vi "test Export SLSC-12252.vi"(8 "error in (no error)":errorcluster, 11 "TestCase in":refnum<class "SLSC Switch Export Unit Tests.lvclass">) -> (0 "error out":errorcluster, 3 "TestCase out":refnum<class "SLSC Switch Export Unit Tests.lvclass">)   [LabVIEW 2017, in "SLSC Switch Export Unit Tests.lvclass"]
uses:
  SLSC Switch Export Unit Tests.lvclass
  <vilib>/NI/NI VeriStand Advanced SysDef API/_Types/SysDef.Export.ctl
  <vilib>/NI/NI VeriStand Advanced SysDef API/_Types/TreeItem.ctl
  <vilib>/NI/NI VeriStand Advanced SysDef API/_Types/TreeItem.Info.ctl
  <vilib>/NI Veristand/Custom Device API/Custom Device Channel.ctl
  <vilib>/NI Veristand/Custom Device API/Custom Device Channel Type.ctl
  <vilib>/NI Veristand/Custom Device API/Custom Device Waveform.ctl
  <vilib>/NI Veristand/Custom Device API/Custom Device Waveform DataType.ctl
  <vilib>/NI/NI VeriStand Advanced SysDef API/_Types/TreeItem.Property.ctl
  SLSC Switch Export Unit Tests.lvclass/SLSC Switch Export Unit Tests.ctl
  <vilib>/addons/_JKI Toolkits/VI Tester/TestCase.llb/TestCase.lvclass
  Scripting/SLSC Switch Scripting.lvlib
  <vilib>/NI/NI VeriStand Custom Device Import and Export Tool/ImportExport.lvlib
  <vilib>/NI/NI VeriStand Advanced SysDef API/SysDef API/Advanced System Definition.lvlib
  <vilib>/NI Veristand/Custom Device API/Custom Device API.lvlib
  C:/Program Files (x86)/National Instruments/LabVIEW 2017/vi.lib/addons/_JKI Toolkits/VI Tester/TestCase.llb/TestCase.lvclass
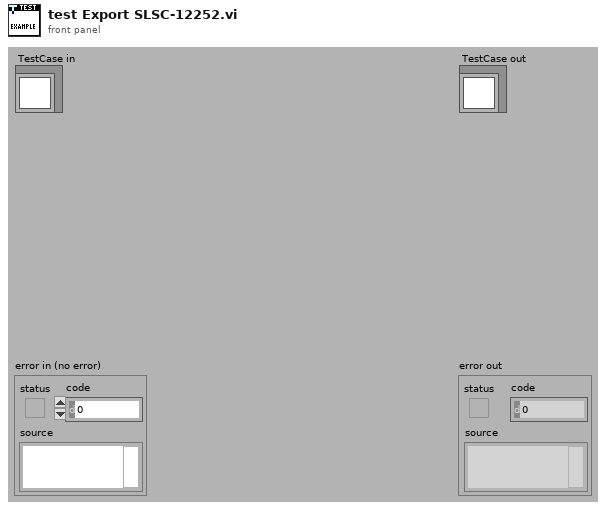
[diagram p1: front panel]
types:
  T1 = typedef "Advanced System Definition.lvlib/SysDef.Export.ctl" = cluster{"Version":string, "Tree":T2[]}
  T2 = typedef "Advanced System Definition.lvlib/TreeItem.ctl" = cluster{"Item Info":T3, "Parent Path":string[], "Properties":T8[]}
  T3 = typedef "Advanced System Definition.lvlib/TreeItem.Info.ctl" = cluster{"Name":string, "Description":string, "GUID":string, "Is Channel":bool, "Channel":T4, "Is Waveform":bool, "Waveform":T6}
  T4 = typedef "Custom Device API.lvlib/Custom Device Channel.ctl" = cluster{"Type":T5, "Units":string, "Default Value":dbl, "Faultable":bool, "Scalable":bool}
  T5 = typedef "Custom Device API.lvlib/Custom Device Channel Type.ctl" = enum16{"Input", "Output"}
  T6 = typedef "Custom Device API.lvlib/Custom Device Waveform.ctl" = cluster{"Data Type":T7, "Units":string}
  T7 = typedef "Custom Device API.lvlib/Custom Device Waveform DataType.ctl" = enum16{"Double", "Complex Double"}
  T8 = typedef "Advanced System Definition.lvlib/TreeItem.Property.ctl" = cluster{"Name":string, "Type":i32, "Value":variant}
  T9 = typedef "Custom Device API.lvlib/Custom Device Item Ref.ctl" = u64
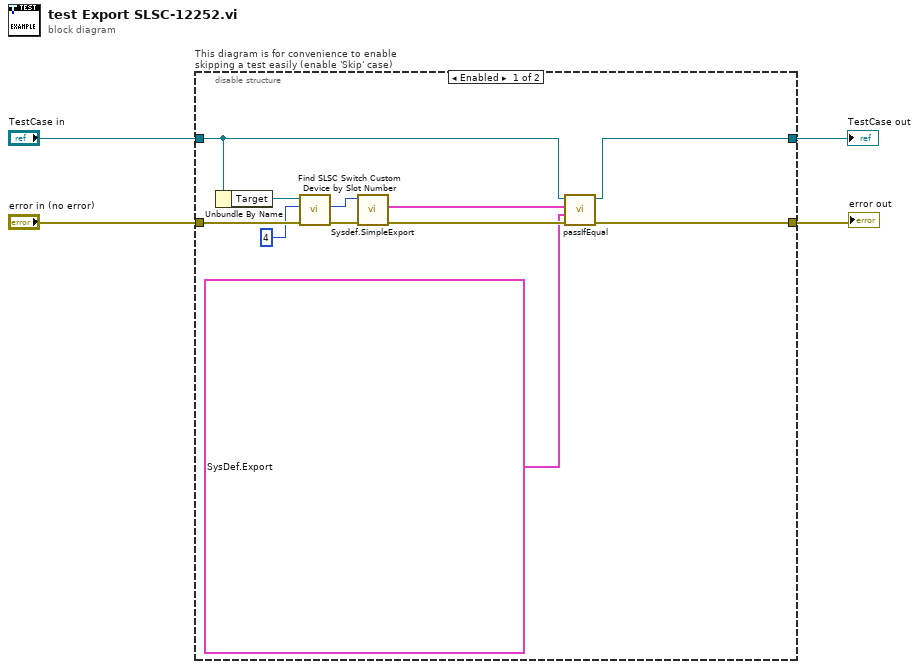
[diagram p0: block diagram]
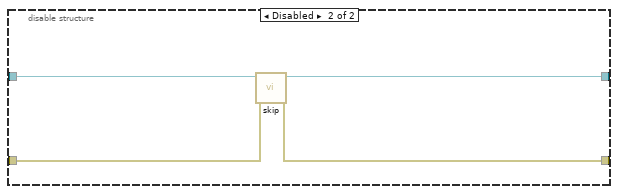
[diagram p2: hidden frame]
diagram:
  n1 = disable-structure "This diagram is for convenience to enable skipping a test easily (enable 'Skip' case)" shown="Enabled" {
    disable-tunnel: "TestCase in" -> [w7 w19]
    disable-tunnel: [w6 w17] -> w1
    disable-tunnel: [w9 w18] -> w3
    disable-tunnel: "error in (no error)" -> [w15 w16]
    frame Enabled {
      n2 = Unbundle By Name(w7) -> ("Target"=w14:refnum<k24>)
      n3 = call "Find SLSC Switch Custom Device by Slot Number.vi"("error in (no error)"=w15, "slot number"=u32 4, "Target in"=w14) -> ("error out"=w12:errorcluster, "SLSC Switch Custom Device Ref"=w11:T9)  [unwired: 6 in, 1 out]
      n4 = call <vilib>:"Sysdef.SimpleExport.vi"("error in (no error)"=w12, "ID"=w11) -> ("error out"=w10:errorcluster, "Export"=w8:T1)  [unwired: 7 in, 1 out]
      n5 = call-dynamic "passIfEqual.vi"("error in (no error)"=w10, "y"=T1 {"Version"="1.0.0", "Tree"=[{"Item Info"={"Name"="Slot 4 (SLSC Switch)", "Description"="", "GUID"="5e47c8de-3ec6-490b-8897-5526d4aea756", "Is Channel"=FALSE, "Channel"={"Type"=enum."Input", "Units"="", "Default Value"=0.0, "Faultable"=FALSE, "Scalable"=FALSE}, "Is Waveform"=FALSE, "Waveform"={"Data Type"=enum."Double", "Units"=""}}, "Parent Path"=["Targets", "Controller", "Hardware", "SLSC", "SLSC Chassis", "Modules"], "Properties"=[{"Name"="user.CD.Routing and Faulting.API Version", "Type"=3, "Value"=variant(u32 1)}, {"Name"="user.CD.Model", "Type"=0, "Value"=variant(string "SLSC-12252", "IsBinary"=variant(bool FALSE))}, {"Name"="user.CD.Routing and Faulting.Resource", "Type"=0, "Value"=variant(string "slsc-12001-0314b282-Mod4", "IsBinary"=variant(bool FALSE))}, {"Name"="user.CD.Topology", "Type"=0, "Value"=variant(string "NI12252_topology", "IsBinary"=variant(bool FALSE))}, {"Name"="user.CD.Capabilities", "Type"=0, "Value"=variant(string "{\"switchesSpecVersion\":1,\"switchesSpecOldestCompatibleVersion\":1,\"relays\":[{\"name\":\"Ch0\",\"actions\":[{\"type\":\"property\",\"resource\":\"Channel_0\",\"value\":\"NI.FIU.Preset.Load\"},{\"type\":\"command\",\"resource\":\"\",\"value\":\"NI.FIU.Update\"}]},{\"name\":\"Ch1\",\"actions\":[{\"type\":\"property\",\"resource\":\"Channel_1\",\"value\":\"NI.FIU.Preset.Load\"},{\"type\":\"command\",\"resource\":\"\",\"value\":\"NI.FIU.Update\"}]},{\"name\":\"Ch2\",\"actions\":[{\"type\":\"property\",\"resource\":\"Channel_2\",\"value\":\"NI.FIU.Preset.Load\"},{\"type\":\"command\",\"resource\":\"\",\"value\":\"NI.FIU.Update\"}]},{\"name\":\"Ch3\",\"actions\":[{\"type\":\"property\",\"resource\":\"Channel_3\",\"value\":\"NI.FIU.Preset.Load\"},{\"type\":\"command\",\"resource\":\"\",\"value\":\"NI.FIU.Update\"}]},{\"name\":\"Ch4\",\"actions\":[{\"type\":\"property\",\"resource\":\"Channel_4\",\"value\":\"NI.FIU.Preset.Load\"},{\"type\":\"command\",\"resource\":\"\",\"value\":\"NI.FIU.Update\"}]},{\"name\":\"Ch5\",\"actions\":[{\"type\":\"property\",\"resource\":\"Channel_5\",\"value\":\"NI.FIU.Preset.Load\"},{\"type\":\"command\",\"resource\":\"\",\"value\":\"NI.FIU.Update\"}]},{\"name\":\"Ch6\",\"actions\":[{\"type\":\"property\",\"resource\":\"Channel_6\",\"value\":\"NI.FIU.Preset.Load\"},{\"type\":\"command\",\"resource\":\"\",\"value\":\"NI.FIU.Update\"}]},{\"name\":\"Ch7\",\"actions\":[{\"type\":\"property\",\"resource\":\"Channel_7\",\"value\":\"NI.FIU.Preset.Load\"},{\"type\":\"command\",\"resource\":\"\",\"value\":\"NI.FIU.Update\"}]},{\"name\":\"Ch0_Ch1\",\"actions\":[{\"type\":\"property\",\"resource\":\"ChannelPair_0\",\"value\":\"NI.FIU.Preset.InterChannel\"},{\"type\":\"command\",\"resource\":\"\",\"value\":\"NI.FIU.Update\"}]},{\"name\":\"Ch2_Ch3\",\"actions\":[{\"type\":\"property\",\"resource\":\"ChannelPair_1\",\"value\":\"NI.FIU.Preset.InterChannel\"},{\"type\":\"command\",\"resource\":\"\",\"value\":\"NI.FIU.Update\"}]},{\"name\":\"Ch4_Ch5\",\"actions\":[{\"type\":\"property\",\"resource\":\"ChannelPair_2\",\"value\":\"NI.FIU.Preset.InterChannel\"},{\"type\":\"command\",\"resource\":\"\",\"value\":\"NI.FIU.Update\"}]},{\"name\":\"Ch6_Ch7\",\"actions\":[{\"type\":\"property\",\"resource\":\"ChannelPair_3\",\"value\":\"NI.FIU.Preset.InterChannel\"},{\"type\":\"command\",\"resource\":\"\",\"value\":\"NI.FIU.Update\"}]}],\"multiStateRelays\":[{\"name\":\"Ch0_Bus\",\"relays\":[{\"name\":\"Ch0_BusA\",\"actions\":[{\"type\":\"property\",\"resource\":\"Channel_0\",\"value\":\"NI.FIU.Preset.BusSource\",\"close\":1},{\"type\":\"command\",\"resource\":\"\",\"value\":\"NI.FIU.Update\"}]},{\"name\":\"Ch0_BusB\",\"actions\":[{\"type\":\"property\",\"resource\":\"Channel_0\",\"value\":\"NI.FIU.Preset.BusSource\",\"close\":2},{\"type\":\"command\",\"resource\":\"\",\"value\":\"NI.FIU.Update\"}]}]},{\"name\":\"Ch1_Bus\",\"relays\":[{\"name\":\"Ch1_BusA\",\"actions\":[{\"type\":\"property\",\"resource\":\"Channel_1\",\"value\":\"NI.FIU.Preset.BusSource\",\"close\":1},{\"type\":\"command\",\"resource\":\"\",\"value\":\"NI.FIU.Update\"}]},{\"name\":\"Ch1_BusB\",\"actions\":[{\"type\":\"property\",\"resource\":\"Channel_1\",\"value\":\"NI.FIU.Preset.BusSource\",\"close\":2},{\"type\":\"command\",\"resource\":\"\",\"value\":\"NI.FIU.Update\"}]}]},{\"name\":\"Ch2_Bus\",\"relays\":[{\"name\":\"Ch2_BusA\",\"actions\":[{\"type\":\"property\",\"resource\":\"Channel_2\",\"value\":\"NI.FIU.Preset.BusSource\",\"close\":1},{\"type\":\"command\",\"resource\":\"\",\"value\":\"NI.FIU.Update\"}]},{\"name\":\"Ch2_BusB\",\"actions\":[{\"type\":\"property\",\"resource\":\"Channel_2\",\"value\":\"NI.FIU.Preset.BusSource\",\"close\":2},{\"type\":\"command\",\"resource\":\"\",\"value\":\"NI.FIU.Update\"}]}]},{\"name\":\"Ch3_Bus\",\"relays\":[{\"name\":\"Ch3_BusA\",\"actions\":[{\"type\":\"property\",\"resource\":\"Channel_3\",\"value\":\"NI.FIU.Preset.BusSource\",\"close\":1},{\"type\":\"command\",\"resource\":\"\",\"value\":\"NI.FIU.Update\"}]},{\"name\":\"Ch3_BusB\",\"actions\":[{\"type\":\"property\",\"resource\":\"Channel_3\",\"value\":\"NI.FIU.Preset.BusSource\",\"close\":2},{\"type\":\"command\",\"resource\":\"\",\"value\":\"NI.FIU.Update\"}]}]},{\"name\":\"Ch4_Bus\",\"relays\":[{\"name\":\"Ch4_BusA\",\"actions\":[{\"type\":\"property\",\"resource\":\"Channel_4\",\"value\":\"NI.FIU.Preset.BusSource\",\"close\":1},{\"type\":\"command\",\"resource\":\"\",\"value\":\"NI.FIU.Update\"}]},{\"name\":\"Ch4_BusB\",\"actions\":[{\"type\":\"property\",\"resource\":\"Channel_4\",\"value\":\"NI.FIU.Preset.BusSource\",\"close\":2},{\"type\":\"command\",\"resource\":\"\",\"value\":\"NI.FIU.Update\"}]}]},{\"name\":\"Ch5_Bus\",\"relays\":[{\"name\":\"Ch5_BusA\",\"actions\":[{\"type\":\"property\",\"resource\":\"Channel_5\",\"value\":\"NI.FIU.Preset.BusSource\",\"close\":1},{\"type\":\"command\",\"resource\":\"\",\"value\":\"NI.FIU.Update\"}]},{\"name\":\"Ch5_BusB\",\"actions\":[{\"type\":\"property\",\"resource\":\"Channel_5\",\"value\":\"NI.FIU.Preset.BusSource\",\"close\":2},{\"type\":\"command\",\"resource\":\"\",\"value\":\"NI.FIU.Update\"}]}]},{\"name\":\"Ch6_Bus\",\"relays\":[{\"name\":\"Ch6_BusA\",\"actions\":[{\"type\":\"property\",\"resource\":\"Channel_6\",\"value\":\"NI.FIU.Preset.BusSource\",\"close\":1},{\"type\":\"command\",\"resource\":\"\",\"value\":\"NI.FIU.Update\"}]},{\"name\":\"Ch6_BusB\",\"actions\":[{\"type\":\"property\",\"resource\":\"Channel_6\",\"value\":\"NI.FIU.Preset.BusSource\",\"close\":2},{\"type\":\"command\",\"resource\":\"\",\"value\":\"NI.FIU.Update\"}]}]},{\"name\":\"Ch7_Bus\",\"relays\":[{\"name\":\"Ch7_BusA\",\"actions\":[{\"type\":\"property\",\"resource\":\"Channel_7\",\"value\":\"NI.FIU.Preset.BusSource\",\"close\":1},{\"type\":\"command\",\"resource\":\"\",\"value\":\"NI.FIU.Update\"}]},{\"name\":\"Ch7_BusB\",\"actions\":[{\"type\":\"property\",\"resource\":\"Channel_7\",\"value\":\"NI.FIU.Preset.BusSource\",\"close\":2},{\"type\":\"command\",\"resource\":\"\",\"value\":\"NI.FIU.Update\"}]}]}],\"topologies\":[{\"name\":\"NI12252_topology\",\"initialState\":{\"open\":[\"Ch0\",\"Ch0_BusA\",\"Ch0_BusB\",\"Ch1\",\"Ch1_BusA\",\"Ch1_BusB\",\"Ch2\",\"Ch2_BusA\",\"Ch2_BusB\",\"Ch3\",\"Ch3_BusA\",\"Ch3_BusB\",\"Ch4\",\"Ch4_BusA\",\"Ch4_BusB\",\"Ch5\",\"Ch5_BusA\",\"Ch5_BusB\",\"Ch6\",\"Ch6_BusA\",\"Ch6_BusB\",\"Ch7\",\"Ch7_BusA\",\"Ch7_BusB\",\"Ch0_Ch1\",\"Ch2_Ch3\",\"Ch4_Ch5\",\"Ch6_Ch7\"],\"close\":[]},\"channelList\":{\"names\":[\"DUT_Ch0\",\"LOAD_Ch0\",\"DUT_Ch1\",\"LOAD_Ch1\",\"DUT_Ch2\",\"LOAD_Ch2\",\"DUT_Ch3\",\"LOAD_Ch3\",\"DUT_Ch4\",\"LOAD_Ch4\",\"DUT_Ch5\",\"LOAD_Ch5\",\"DUT_Ch6\",\"LOAD_Ch6\",\"DUT_Ch7\",\"LOAD_Ch7\",\"BusA\",\"BusB\"]},\"connectionList\":[{\"src\":\"DUT_Ch0\",\"dest\":\"LOAD_Ch0\",\"relays\":[\"Ch0\"]},{\"src\":\"DUT_Ch0\",\"dest\":\"BusA\",\"relays\":[\"Ch0_BusA\"]},{\"src\":\"DUT_Ch0\",\"dest\":\"BusB\",\"relays\":[\"Ch0_BusB\"]},{\"src\":\"DUT_Ch1\",\"dest\":\"LOAD_Ch1\",\"relays\":[\"Ch1\"]},{\"src\":\"DUT_Ch1\",\"dest\":\"BusA\",\"relays\":[\"Ch1_BusA\"]},{\"src\":\"DUT_Ch1\",\"dest\":\"BusB\",\"relays\":[\"Ch1_BusB\"]},{\"src\":\"DUT_Ch2\",\"dest\":\"LOAD_Ch2\",\"relays\":[\"Ch2\"]},{\"src\":\"DUT_Ch2\",\"dest\":\"BusA\",\"relays\":[\"Ch2_BusA\"]},{\"src\":\"DUT_Ch2\",\"dest\":\"BusB\",\"relays\":[\"Ch2_BusB\"]},{\"src\":\"DUT_Ch3\",\"dest\":\"LOAD_Ch3\",\"relays\":[\"Ch3\"]},{\"src\":\"DUT_Ch3\",\"dest\":\"BusA\",\"relays\":[\"Ch3_BusA\"]},{\"src\":\"DUT_Ch3\",\"dest\":\"BusB\",\"relays\":[\"Ch3_BusB\"]},{\"src\":\"DUT_Ch4\",\"dest\":\"LOAD_Ch4\",\"relays\":[\"Ch4\"]},{\"src\":\"DUT_Ch4\",\"dest\":\"BusA\",\"relays\":[\"Ch4_BusA\"]},{\"src\":\"DUT_Ch4\",\"dest\":\"BusB\",\"relays\":[\"Ch4_BusB\"]},{\"src\":\"DUT_Ch5\",\"dest\":\"LOAD_Ch5\",\"relays\":[\"Ch5\"]},{\"src\":\"DUT_Ch5\",\"dest\":\"BusA\",\"relays\":[\"Ch5_BusA\"]},{\"src\":\"DUT_Ch5\",\"dest\":\"BusB\",\"relays\":[\"Ch5_BusB\"]},{\"src\":\"DUT_Ch6\",\"dest\":\"LOAD_Ch6\",\"relays\":[\"Ch6\"]},{\"src\":\"DUT_Ch6\",\"dest\":\"BusA\",\"relays\":[\"Ch6_BusA\"]},{\"src\":\"DUT_Ch6\",\"dest\":\"BusB\",\"relays\":[\"Ch6_BusB\"]},{\"src\":\"DUT_Ch7\",\"dest\":\"LOAD_Ch7\",\"relays\":[\"Ch7\"]},{\"src\":\"DUT_Ch7\",\"dest\":\"BusA\",\"relays\":[\"Ch7_BusA\"]},{\"src\":\"DUT_Ch7\",\"dest\":\"BusB\",\"relays\":[\"Ch7_BusB\"]},{\"src\":\"DUT_Ch0\",\"dest\":\"DUT_Ch1\",\"relays\":[\"Ch0_Ch1\"]},{\"src\":\"DUT_Ch2\",\"dest\":\"DUT_Ch3\",\"relays\":[\"Ch2_Ch3\"]},{\"src\":\"DUT_Ch4\",\"dest\":\"DUT_Ch5\",\"relays\":[\"Ch4_Ch5\"]},{\"src\":\"DUT_Ch6\",\"dest\":\"DUT_Ch7\",\"relays\":[\"Ch6_Ch7\"]}],\"muxList\":[{\"src\":\"DUT_Ch0\",\"dest\":[\"BusA\",\"BusB\"]},{\"src\":\"DUT_Ch1\",\"dest\":[\"BusA\",\"BusB\"]},{\"src\":\"DUT_Ch2\",\"dest\":[\"BusA\",\"BusB\"]},{\"src\":\"DUT_Ch3\",\"dest\":[\"BusA\",\"BusB\"]},{\"src\":\"DUT_Ch4\",\"dest\":[\"BusA\",\"BusB\"]},{\"src\":\"DUT_Ch5\",\"dest\":[\"BusA\",\"BusB\"]},{\"src\":\"DUT_Ch6\",\"dest\":[\"BusA\",\"BusB\"]},{\"src\":\"DUT_Ch7\",\"dest\":[\"BusA\",\"BusB\"]}]}]}", "IsBinary"=variant(bool FALSE))}, {"Name"="user.CD.Slot #", "Type"=2, "Value"=variant(i32 4)}]}, {"Item Info"={"Name"="Endpoint Configuration", "Description"="", "GUID"="f35fa8c0-605e-4a68-bbe7-65ff21f249ff", "Is Channel"=FALSE, "Channel"={"Type"=enum."Input", "Units"="", "Default Value"=0.0, "Faultable"=FALSE, "Scalable"=FALSE}, "Is Waveform"=FALSE, "Waveform"={"Data Type"=enum."Double", "Units"=""}}, "Parent Path"=["Targets", "Controller", "Hardware", "SLSC", "SLSC Chassis", "Modules", "Slot 4 (SLSC Switch)"], "Properties"=[{"Name"="user.CD.DUT_Ch0", "Type"=0, "Value"=variant(string "Load", "IsBinary"=variant(bool FALSE))}, {"Name"="user.CD.LOAD_Ch0", "Type"=0, "Value"=variant(string "Load", "IsBinary"=variant(bool FALSE))}, {"Name"="user.CD.DUT_Ch1", "Type"=0, "Value"=variant(string "Load", "IsBinary"=variant(bool FALSE))}, {"Name"="user.CD.LOAD_Ch1", "Type"=0, "Value"=variant(string "Load", "IsBinary"=variant(bool FALSE))}, {"Name"="user.CD.DUT_Ch2", "Type"=0, "Value"=variant(string "Load", "IsBinary"=variant(bool FALSE))}, {"Name"="user.CD.LOAD_Ch2", "Type"=0, "Value"=variant(string "Load", "IsBinary"=variant(bool FALSE))}, {"Name"="user.CD.DUT_Ch3", "Type"=0, "Value"=variant(string "Load", "IsBinary"=variant(bool FALSE))}, {"Name"="user.CD.LOAD_Ch3", "Type"=0, "Value"=variant(string "Load", "IsBinary"=variant(bool FALSE))}, {"Name"="user.CD.DUT_Ch4", "Type"=0, "Value"=variant(string "Load", "IsBinary"=variant(bool FALSE))}, {"Name"="user.CD.LOAD_Ch4", "Type"=0, "Value"=variant(string "Load", "IsBinary"=variant(bool FALSE))}, {"Name"="user.CD.DUT_Ch5", "Type"=0, "Value"=variant(string "Load", "IsBinary"=variant(bool FALSE))}, {"Name"="user.CD.LOAD_Ch5", "Type"=0, "Value"=variant(string "Load", "IsBinary"=variant(bool FALSE))}, {"Name"="user.CD.DUT_Ch6", "Type"=0, "Value"=variant(string "Load", "IsBinary"=variant(bool FALSE))}, {"Name"="user.CD.LOAD_Ch6", "Type"=0, "Value"=variant(string "Load", "IsBinary"=variant(bool FALSE))}, {"Name"="user.CD.DUT_Ch7", "Type"=0, "Value"=variant(string "Load", "IsBinary"=variant(bool FALSE))}, {"Name"="user.CD.LOAD_Ch7", "Type"=0, "Value"=variant(string "Load", "IsBinary"=variant(bool FALSE))}, {"Name"="user.CD.BusA", "Type"=0, "Value"=variant(string "Load", "IsBinary"=variant(bool FALSE))}, {"Name"="user.CD.BusB", "Type"=0, "Value"=variant(string "Load", "IsBinary"=variant(bool FALSE))}]}, {"Item Info"={"Name"="Status", "Description"="", "GUID"="80DE2635-1DC5-B67A-CA46-E31C1EC1F9C0", "Is Channel"=FALSE, "Channel"={"Type"=enum."Input", "Units"="", "Default Value"=0.0, "Faultable"=FALSE, "Scalable"=FALSE}, "Is Waveform"=FALSE, "Waveform"={"Data Type"=enum."Double", "Units"=""}}, "Parent Path"=["Targets", "Controller", "Hardware", "SLSC", "SLSC Chassis", "Modules", "Slot 4 (SLSC Switch)"], "Properties"=[]}, {"Item Info"={"Name"="Status code", "Description"="Status code of the custom device. A negative value indicates failure. A positive value indicates warning.", "GUID"="03D3BB99-1485-13A6-561D1F898F032919", "Is Channel"=TRUE, "Channel"={"Type"=enum."Output", "Units"="", "Default Value"=0.0, "Faultable"=FALSE, "Scalable"=FALSE}, "Is Waveform"=FALSE, "Waveform"={"Data Type"=enum."Double", "Units"=""}}, "Parent Path"=["Targets", "Controller", "Hardware", "SLSC", "SLSC Chassis", "Modules", "Slot 4 (SLSC Switch)", "Status"], "Properties"=[]}, {"Item Info"={"Name"="Heartbeat", "Description"="Running count used for debugging. If this channel continues to increment, the custom device is still executing.", "GUID"="03D3BB99-1485-13A6-561D1F898F032919", "Is Channel"=TRUE, "Channel"={"Type"=enum."Output", "Units"="", "Default Value"=0.0, "Faultable"=FALSE, "Scalable"=FALSE}, "Is Waveform"=FALSE, "Waveform"={"Data Type"=enum."Double", "Units"=""}}, "Parent Path"=["Targets", "Controller", "Hardware", "SLSC", "SLSC Chassis", "Modules", "Slot 4 (SLSC Switch)", "Status"], "Properties"=[]}]} ("Export"), "x"=w8, "TestCase in"=w7) -> ("error out"=w9:errorcluster, "TestCase out"=w6:refnum<class "SLSC Switch Export Unit Tests.lvclass">)  [unwired: 6 in]
    }
    frame Disabled {
      # "skip test result while test is under development"
      n6 = call <vilib>:"skip.vi"("error in (no error)"=w16, "TestCase in"=w19) -> ("error out"=w18:errorcluster, "TestCase out"=w17:refnum<class "SLSC Switch Export Unit Tests.lvclass">)  [unwired: 8 in]
    }
  }
  "error out" <- w3
  "TestCase out" <- w1
